vi "(SUBVI) - Ultra.vi"(9 "Port (Port 1)":T2 items=["Port 1", "Port 2", "Port 3", "Port 4"], 11 "NXT/EV3":T1) -> (0 "Inches":sgl, 3 "NXT/EV3 2":T1)   [LabVIEW 2016, in "testrobot.lvrbt"]
uses:
  testrobot.lvrbt
  <vilib>/NXT/Subs/LVHSConnector.ctl
  <vilib>/NXT/LegoClasses/BrickReference/BrickReference.lvclass
  <vilib>/NXT/Block Support/NXT_InputPort.ctl
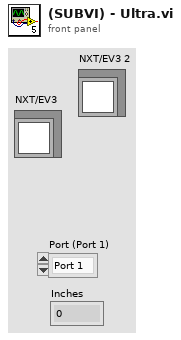
[diagram p1: front panel]
types:
  T1 = typedef "LVHSConnector.ctl" = refnum<class "BrickReference.lvclass">
  T2 = typedef "NXT_InputPort.ctl" = u32
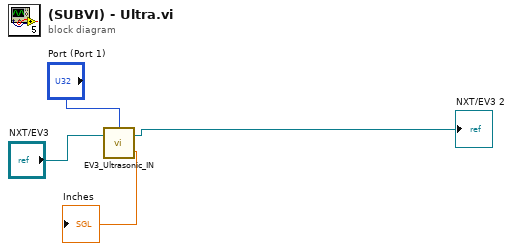
[diagram p0: block diagram]
diagram:
  n1 = call <vilib>:"EV3_Ultrasonic_IN.vi"("NXT/EV3"="NXT/EV3", "Port (Port 1)"="Port (Port 1)") -> ("Inches"=→"Inches":sgl, "NXT/EV3"=→"NXT/EV3 2":T1)  [unwired: 1 in]
